vi "applyPulseFinsihToDevice.vi"(8 "error in (no error)":errorcluster, 10 "device":refnum<class "device.lvclass">, 11 "ScriptListCompiler in":refnum<class "ScriptListCompiler.lvclass">) -> (0 "error out":errorcluster, 2 "device out":refnum<class "device.lvclass">, 3 "ScriptListCompiler out":refnum<class "ScriptListCompiler.lvclass">)   [LabVIEW 2011, in "Compiler.lvlib" / "ScriptListCompiler.lvclass"]
uses:
  ScriptListCompiler.lvclass
  DatabaseHelpers/Database Objects/device/device.lvclass
  Scripting/ScriptingEvent/ScriptEventList/ScriptEventList.lvclass
panel:
  # "this calibrates too."
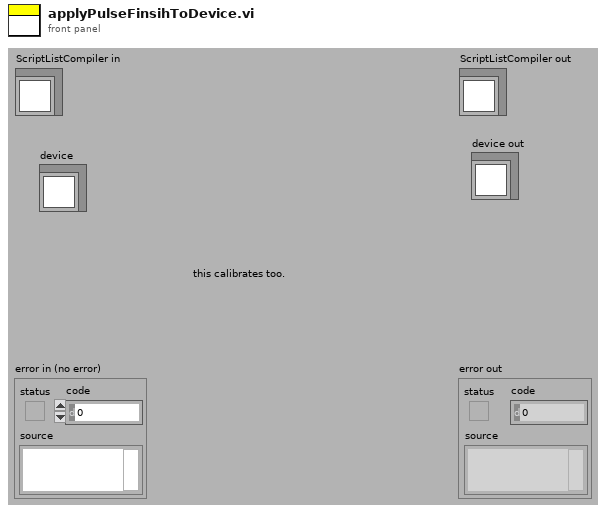
[diagram p1: front panel]
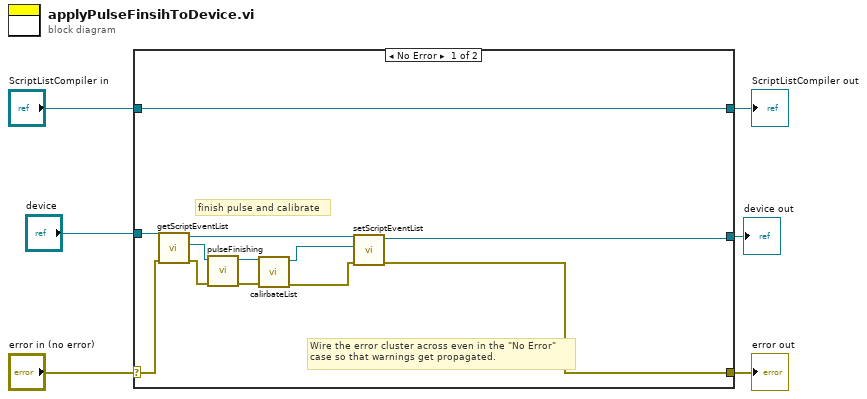
[diagram p0: block diagram]
diagram:
  n1 = case shown="No Error" "error in (no error)" {
    selector: "error in (no error)" -> [w16 w20]
    tunnel: [w7 w20] -> w5
    tunnel: [w18 w19] -> w3
    tunnel: "ScriptListCompiler in" -> [w18 w19]
    tunnel: "device" -> [w17 _]
    tunnel: [w12 _] -> w1
    frame No Error {
      # "finish pulse and calibrate"
      # "Wire the error cluster across even in the \"No Error\"\ncase so that warnings get propagated."
      n2 = call "getScriptEventList.vi"("error in (no error)"=w16, "device.lvclass in"=w17) -> ("error out"=w13:errorcluster, "ScriptEventList"=w14:refnum<class "ScriptEventList.lvclass">, "device.lvclass out"=w15:refnum<class "device.lvclass">)  [unwired: 7 in]
      n3 = call "pulseFinishing.vi"("error in (no error)"=w13, "ScriptEventList in"=w14) -> ("error out"=w10:errorcluster, "ScriptEventList out"=w11:refnum<class "ScriptEventList.lvclass">)  [unwired: 8 in]
      n4 = call "calirbateList.vi"("error in (no error)"=w10, "ScriptEventList in"=w11) -> ("error out"=w9:errorcluster, "ScriptEventList out"=w8:refnum<class "ScriptEventList.lvclass">)  [unwired: 8 in]
      n5 = call "setScriptEventList.vi"("error in (no error)"=w9, "ScriptEventList"=w8, "device.lvclass in"=w15) -> ("error out"=w7:errorcluster, "device.lvclass out"=w12:refnum<class "device.lvclass">)  [unwired: 7 in]
    }
    frame Error {
    }
  }
  "error out" <- w5
  "ScriptListCompiler out" <- w3
  "device out" <- w1
